vi "TORC-TapeMeasureTeleop.vi"(8 "Speed":dbl=0.5, 10 "Reverse?":bool, 11 "Forward?":bool) -> ()   [LabVIEW 2014]
doc: "One of the VIs created by TORC 2137 to control the tape measure. Place this within your code's Teleop.vi.\n\nThere are two required inputs; one tells whether the tape measure should move forward, and one tells whether it should move backwards. If both buttons are pressed simultaneously, the inputs will negate each other and the tape measure will not move.\n\nThere is an optional input for the speed, which is a decimal value from 1 to -1, that gives the speed; the default is 0.5."
uses:
  TORC-TapeMeasureGlobal.vi
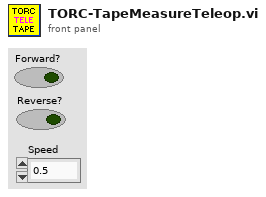
[diagram p1: front panel]
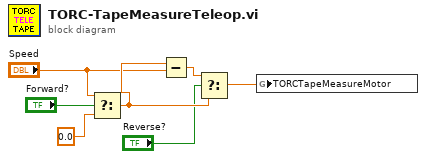
[diagram p0: block diagram]
diagram:
  n1 = Select(t="Speed", s="Forward?", f=0.0) -> (s? t:f=w5:dbl)
  n2 = Subtract(x=w5, y="Speed") -> (x-y=w7:dbl)
  n3 = Select(t=w7, s="Reverse?", f=w5) -> (s? t:f=w3:dbl)
  n4 = global write "TORC-TapeMeasureGlobal.vi" "TORCTapeMeasureMotor"(w3) -> ()
